vi "main.vi"() -> ()   [LabVIEW 2016, in "AIRMAR WeatherCaster.lvlib"]
uses:
  AIRMAR WeatherCaster.lvlib
  <vilib>/Utility/miscctls.llb/LVPointTypeDef.ctl
  NMEA serial.vi
  WXA100-06MH.vi
  <vilib>/Utility/config.llb/NI_LVConfig.lvlib
panel:
  in  "锁":bool
  in  "型号变更":bool
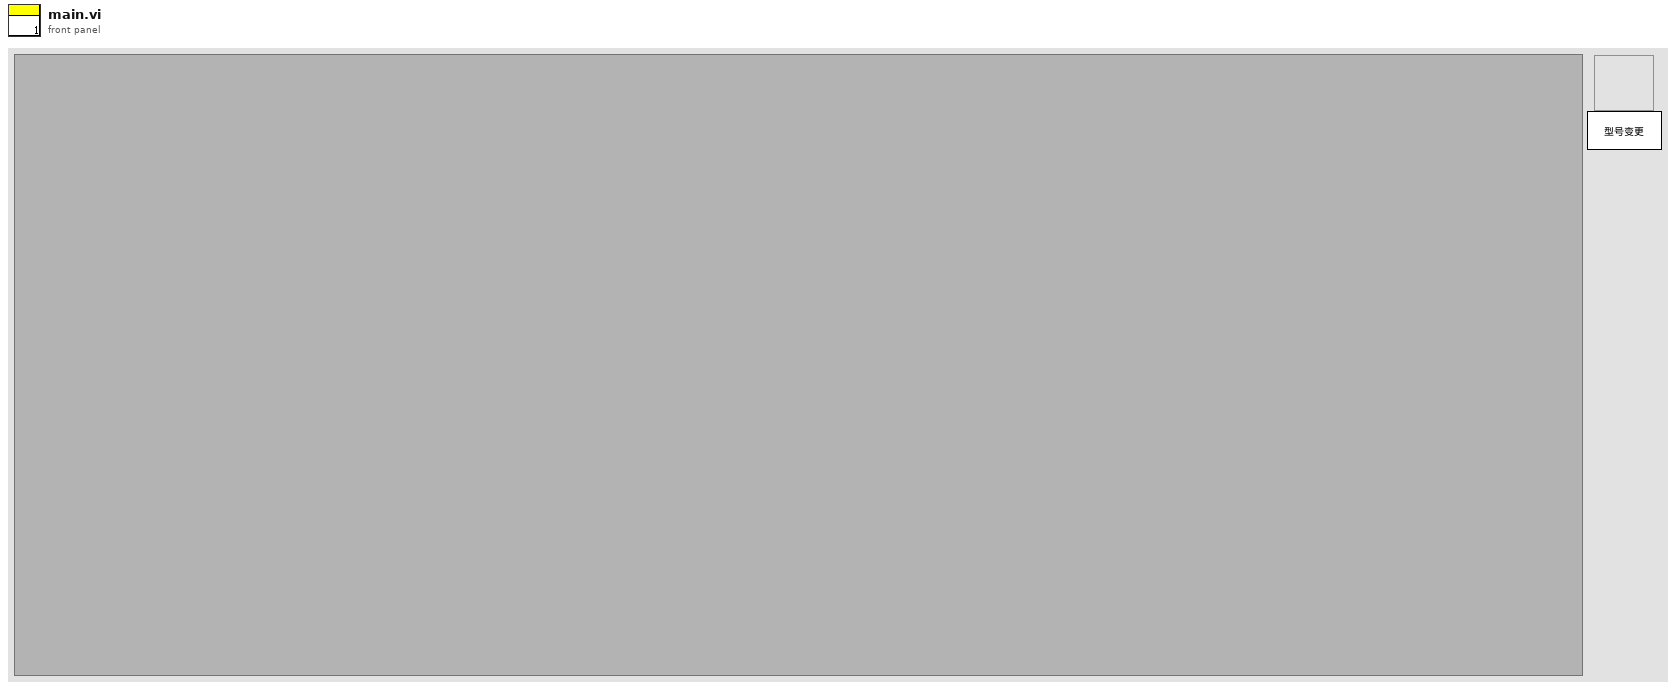
[diagram p1: front panel]
types:
  T1 = typedef "LVPointTypeDef.ctl" = cluster{"Horizontal":i16, "Vertical":i16}
  T2 = typedef "NI_LVConfig.lvlib/Config Data RefNum.ctl" = refnum<k1>
  T3 = enum32{"Bad", "Idle", "Run top level", "Running"}
  T4 = cluster{"确定":bool, "单选按钮":enum32{"NMEA", "WXA100"}}
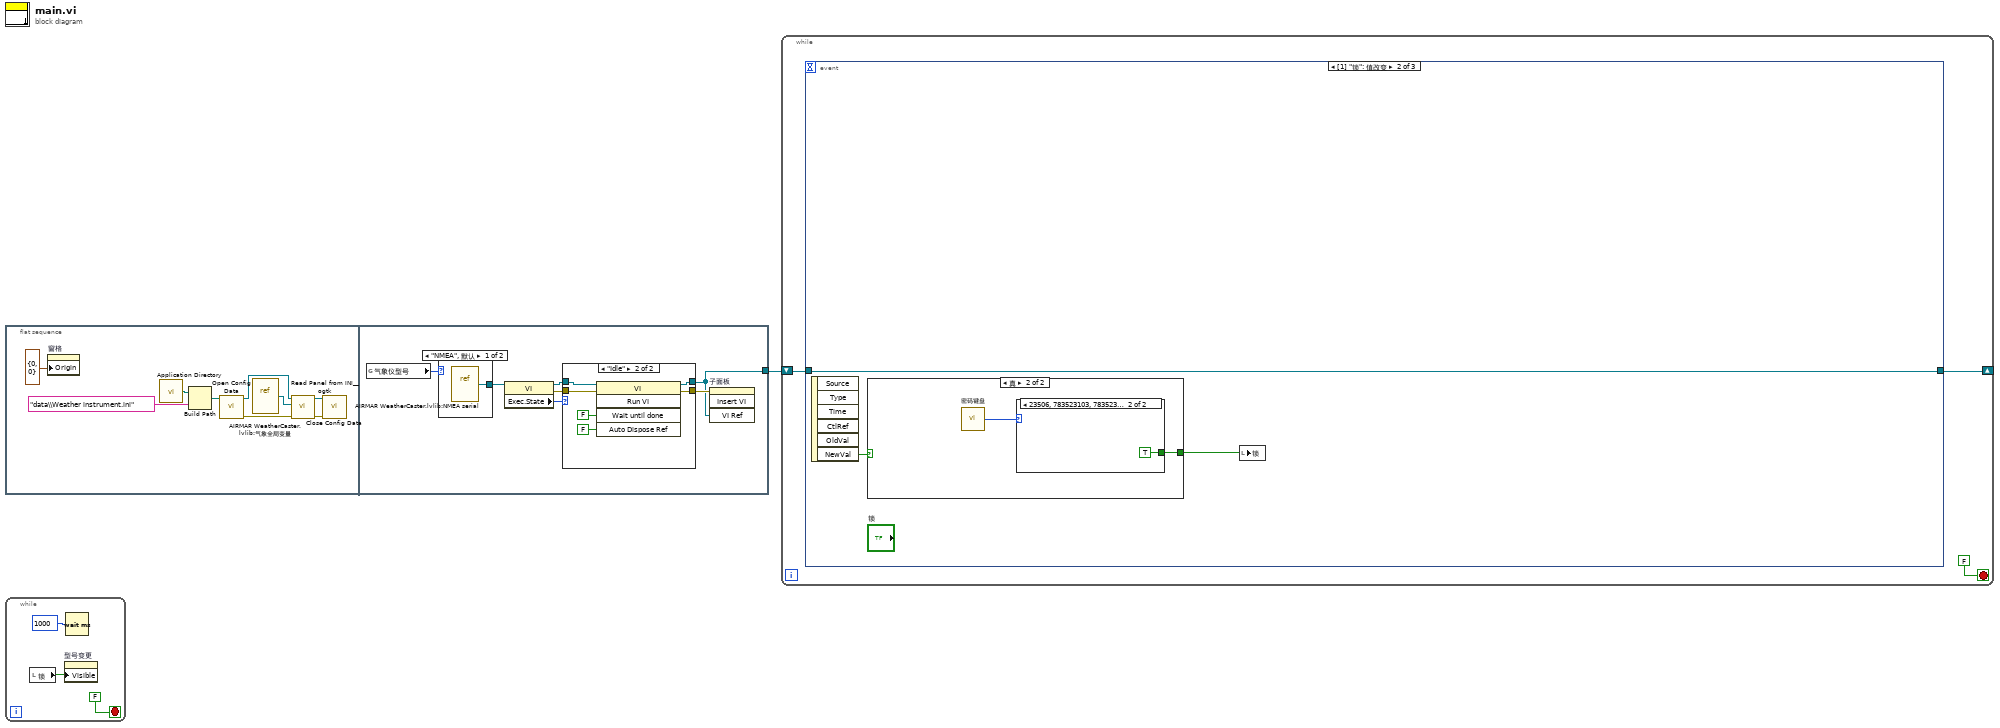
[diagram p0: block diagram]
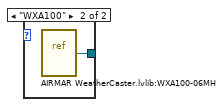
[diagram p3: hidden frame]
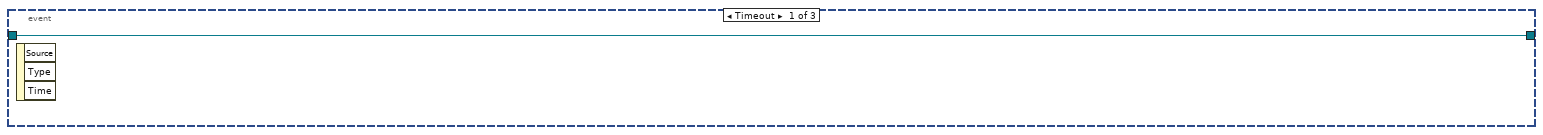
[diagram p4: hidden frame]
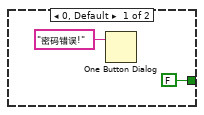
[diagram p6: hidden frame]
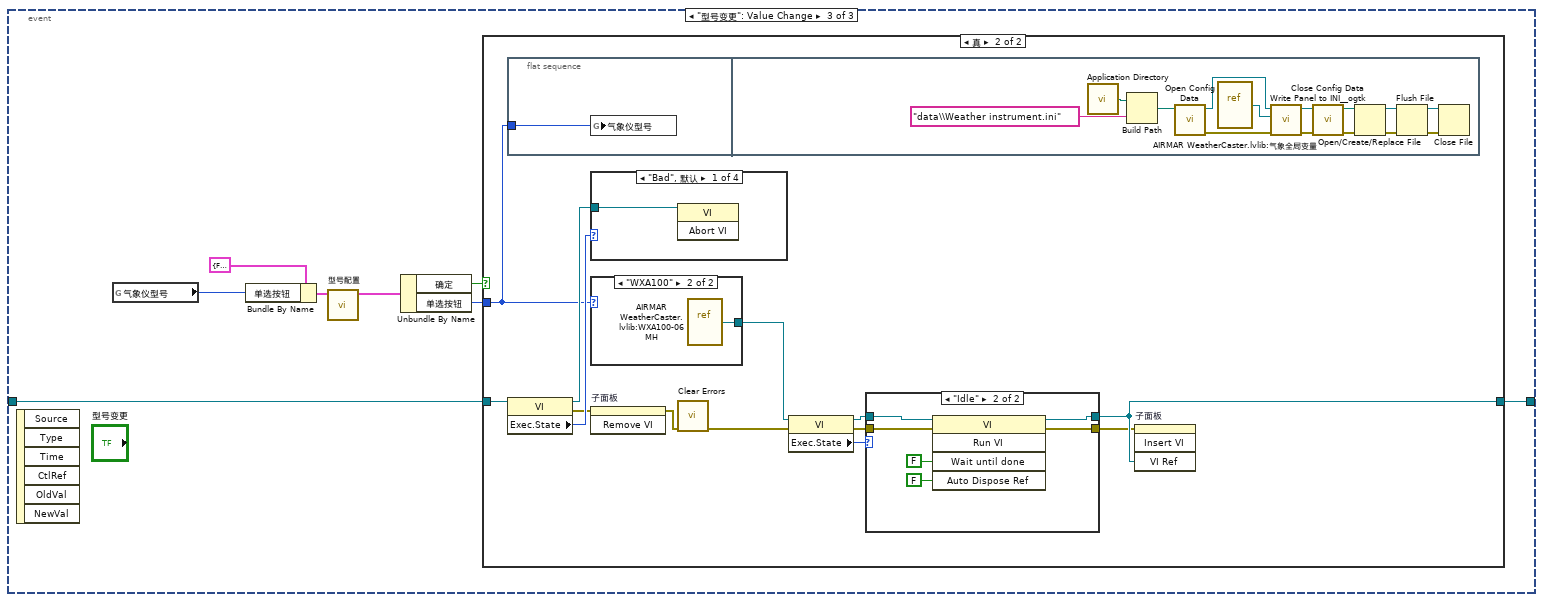
[diagram p7: hidden frame]
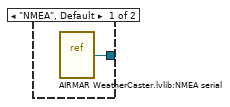
[diagram p9: hidden frame]
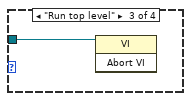
[diagram p11: hidden frame]
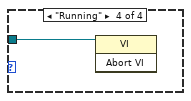
[diagram p12: hidden frame]
diagram:
  n1 = flat-sequence {
    tunnel: [w11] -> w1
    frame #0 {
      n2 = property on="窗格" class="Pane"("Origin"=T1 {"Horizontal"=0, "Vertical"=0} ("原点")) -> ()  [unwired: 2 in, 2 out]
      n3 = call <vilib>:"Application Directory.vi"() -> ("Application Directory"=w3:path)
      n4 = Build Path(base path=w3, name or relative path="data\\Weather instrument.ini" ("名称或相对路径")) -> (appended path=w5:path)
      n5 = call <vilib>:"Open Config Data.vi"("configuration file path"=w5) -> ("error out"=w9:errorcluster, "refnum"=w6:T2)  [unwired: 8 in, 1 out]
      n6 = vi-ref "AIRMAR WeatherCaster.lvlib:气象全局变量.vi"() -> (w7:refnum<vi>)
      n7 = call <userlib>:"Read Panel from INI__ogtk.vi"("error in (no error)"=w9, "VI ref"=w7, "refnum"=w6) -> ("error out"=w10:errorcluster, "refnum out"=w8:T2)  [unwired: 7 in]
      n8 = call <vilib>:"Close Config Data.vi"("error in (no error)"=w10, "refnum"=w8) -> ()  [unwired: 8 in, 2 out]
    }
    frame #1 {
      n9 = global read "气象全局变量.vi" "气象仪型号"() -> (w17:enum16{"NMEA", "WXA100"})
      n10 = case shown="\"NMEA\", 默认" w17 {
        tunnel: [w26 w27] -> w13
        frame "NMEA", Default {
          n11 = vi-ref "AIRMAR WeatherCaster.lvlib:NMEA serial.vi"() -> (w26:refnum<vi>)
        }
        frame "WXA100" {
          n12 = vi-ref "AIRMAR WeatherCaster.lvlib:WXA100-06MH.vi"() -> (w27:refnum<vi>)
        }
      }
      n13 = property class="VI"(reference=w13) -> (reference out=w15:refnum<vi>, error out=w14:errorcluster, "Exec.State"=w16:T3)  [unwired: 1 in]
      n14 = case shown="\"Idle\"" w16 {
        tunnel: w15 -> [w19 w25]
        tunnel: [w19 w22] -> w11
        tunnel: w14 -> [w18 w21]
        tunnel: [w18 w20] -> w12
        frame "Bad", Default {
        }
        frame "Idle" {
          n15 = invoke class="VI" method="Run VI"(reference=w25, error in=w21, "Wait until done"=FALSE ("结束前等待"), "Auto Dispose Ref"=FALSE ("自动销毁引用")) -> (reference out=w22:refnum<vi>, error out=w20:errorcluster)  [unwired: 1 in, 3 out]
        }
      }
      n16 = invoke on="子面板" class="SubPnl" method="Insert VI"(error in=w12, "VI Ref"=w11) -> ()  [unwired: 2 in, 4 out]
    }
  }
  n17 = while {
    stop <- FALSE stop-if-true
    n18 = local read "锁"() -> (w28:bool)
    n19 = property on="型号变更" class="Bool"("Visible"=w28) -> ()  [unwired: 2 in, 2 out]
    n20 = Wait (ms)(milliseconds to wait=u32 1000 ("等待时间（毫秒）")) -> ()  [unwired: 1 out]
  }
  n21 = while {
    shift-right: [w31] -> _
    shift-left: w1 -> [w32]
    stop <- FALSE stop-if-true
    n22 = event shown="[1] \"锁\": 值改变" {
      selector: _ -> [_ _ _]
      dyn-events: _ -> [_ _ _]
      timeout: _ -> [_ _ _]
      tunnel: w32 -> [w34 w35 w45]
      tunnel: [w34 w35 w44] -> w31
      event Timeout {
        n23 = event-data() -> ()  [unwired: 1 in, 3 out]
      }
      event "锁": Value Change {
        n24 = event-data() -> ("NewVal"=w37:bool)  [unwired: 1 in, 5 out]
        n25 = case shown="真" w37 {
          selector: w37 -> [w38 _]
          tunnel: [w38 w39] -> w36
          frame False {
          }
          frame True {
            n26 = call "密码键盘.vi"() -> ("NewNumber"=w40:u32)  [unwired: 1 in]
            n27 = case shown="23506, 783523103, 783523506" w40 {
              tunnel: [FALSE TRUE] -> w39
              frame 0, Default {
                n28 = One Button Dialog(message="密码错误!" ("消息")) -> ()  [unwired: 1 in, 1 out]
              }
              frame 23506, 783523103, 783523506 {
              }
            }
          }
        }
        n29 = local write "锁"(w36) -> ()
      }
      event "型号变更": Value Change {
        n30 = event-data() -> ()  [unwired: 1 in, 6 out]
        n31 = global read "气象全局变量.vi" "气象仪型号"() -> (w50:enum16{"NMEA", "WXA100"})
        n32 = Bundle By Name(cluster=T4 {"确定"=FALSE, "单选按钮"=enum."WXA100"} ("输入"), "单选按钮"=w50) -> (w49:T4)
        n33 = call "型号配置.vi"("输入"=w49) -> ("输出"=w48:T4)  [unwired: 10 in]
        n34 = Unbundle By Name(w48) -> ("确定"=w47:bool, "单选按钮"=w46:enum32{"NMEA", "WXA100"})
        n35 = case shown="真" w47 {
          tunnel: w46 -> [_ w58]
          tunnel: w45 -> [w52 w57]
          tunnel: [w52 w56] -> w44
          frame False {
          }
          frame True {
            n36 = flat-sequence {
              tunnel: w58 -> [w79]
              frame #0 {
                n37 = global write "气象全局变量.vi" "气象仪型号"(w79) -> ()
              }
              frame #1 {
                n38 = call <vilib>:"Application Directory.vi"() -> ("Application Directory"=w92:path)
                n39 = Build Path(base path=w92, name or relative path="data\\Weather instrument.ini" ("名称或相对路径")) -> (appended path=w91:path)
                n40 = call <vilib>:"Open Config Data.vi"("configuration file path"=w91) -> ("error out"=w88:errorcluster, "refnum"=w90:T2)  [unwired: 8 in, 1 out]
                n41 = vi-ref "AIRMAR WeatherCaster.lvlib:气象全局变量.vi"() -> (w93:refnum<vi>)
                n42 = call <userlib>:"Write Panel to INI__ogtk.vi"("error in (no error)"=w88, "VI ref"=w93, "refnum"=w90) -> ("error out"=w87:errorcluster, "refnum out"=w89:T2)  [unwired: 7 in]
                n43 = call <vilib>:"Close Config Data.vi"("error in (no error)"=w87, "refnum"=w89) -> ("error out"=w82:errorcluster, "file path"=w81:path)  [unwired: 8 in]
                n44 = Open/Create/Replace File(file path (use dialog)=w81, error in=w82) -> (refnum out=w85:refnum<file>, error out=w86:errorcluster)  [unwired: 4 in, 1 out]
                n45 = Flush File(refnum=w85, error in=w86) -> (refnum out=w84:refnum<file>, error out=w83:errorcluster)
                n46 = Close File(refnum=w84, error in=w83) -> ()  [unwired: 2 out]
              }
            }
            n47 = property class="VI"(reference=w57) -> (reference out=w63:refnum<vi>, error out=w53:errorcluster, "Exec.State"=w62:T3)  [unwired: 1 in]
            n48 = case shown="\"Bad\", 默认" w62 {
              tunnel: w63 -> [w68 _ w69 w70]
              frame "Bad", Default {
                n49 = invoke class="VI" method="Abort VI"(reference=w68) -> ()  [unwired: 2 in, 3 out]
              }
              frame "Idle" {
              }
              frame "Run top level" {
                n50 = invoke class="VI" method="Abort VI"(reference=w69) -> ()  [unwired: 2 in, 3 out]
              }
              frame "Running" {
                n51 = invoke class="VI" method="Abort VI"(reference=w70) -> ()  [unwired: 2 in, 3 out]
              }
            }
            n52 = case shown="\"WXA100\"" w58 {
              tunnel: [w66 w67] -> w65
              frame "NMEA", Default {
                n53 = vi-ref "AIRMAR WeatherCaster.lvlib:NMEA serial.vi"() -> (w66:refnum<vi>)
              }
              frame "WXA100" {
                n54 = vi-ref "AIRMAR WeatherCaster.lvlib:WXA100-06MH.vi"() -> (w67:refnum<vi>)
              }
            }
            n55 = invoke on="子面板" class="SubPnl" method="Remove VI"(error in=w53) -> (error out=w54:errorcluster)  [unwired: 2 in, 2 out]
            n56 = call <vilib>:"Clear Errors.vi"("error in (no error)"=w54) -> ("error out"=w64:errorcluster)  [unwired: 5 in, 1 out]
            n57 = property class="VI"(reference=w65, error in=w64) -> (reference out=w60:refnum<vi>, error out=w61:errorcluster, "Exec.State"=w59:T3)
            n58 = case shown="\"Idle\"" w59 {
              tunnel: w60 -> [w72 w78]
              tunnel: [w72 w75] -> w56
              tunnel: w61 -> [w71 w74]
              tunnel: [w71 w73] -> w55
              frame "Bad", Default {
              }
              frame "Idle" {
                n59 = invoke class="VI" method="Run VI"(reference=w78, error in=w74, "Wait until done"=FALSE ("结束前等待"), "Auto Dispose Ref"=FALSE ("自动销毁引用")) -> (reference out=w75:refnum<vi>, error out=w73:errorcluster)  [unwired: 1 in, 3 out]
              }
            }
            n60 = invoke on="子面板" class="SubPnl" method="Insert VI"(error in=w55, "VI Ref"=w56) -> ()  [unwired: 2 in, 4 out]
          }
        }
      }
    }
  }
